vi "Tip Strip.vi"(7 "Calling VI's reference":refnum<vi>, 11 "Ref Array":refnum<vi>[](array[refnum])) -> ()   [LabVIEW 2017]
doc: "Registers events for array of references passed in. When a control is moused over, the tip strip text is shown in a popup as long as the mouse os over the control. The tip strip disappears when the mouse leaves the control or the mouse is clicked on the control.\n\nNEEDS: resize the tip strip to size of text."
uses:
  <vilib>/Utility/miscctls.llb/LVRectTypeDef.ctl
  <vilib>/Utility/inputDevices.llb/mouseAcquire.vi
panel:
  in  "Fade-Out Time [150]":u32=150
  in  "Fade-In Time [250]":u32=250
  out "error out":errorcluster
  in  "stop notifier":refnum<notifier>
  out "Custom Tip Strip":string
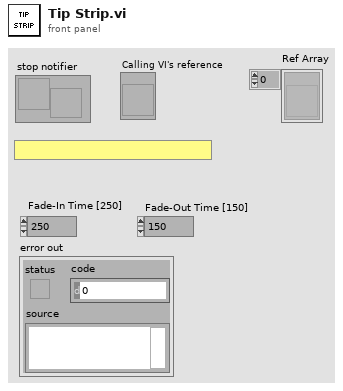
[diagram p1: front panel]
types:
  T1 = typedef "LVPositionTypeDef.ctl" = cluster{"Left":i32, "Top":i32}
  T2 = enum32{"Invalid", "Standard", "Closed", "Hidden", "Minimized", "Maximized"}
  T3 = cluster{"Font Name:":string, "Size":i16, "Strikeout?":bool, "Italic?":bool, "Underline?":bool, "Outline?":bool, "Shadow?":bool, "Bold?":bool}
  T4 = typedef "LVRectTypeDef.ctl" = cluster{"Left":i16, "Top":i16, "Right":i16, "Bottom":i16}
  T5 = cluster{"left":i16, "top":i16, "right":i16, "bottom":i16}
  T6 = cluster{"Horizontal":i32, "Vertical":i32, "Scrolling":i32}
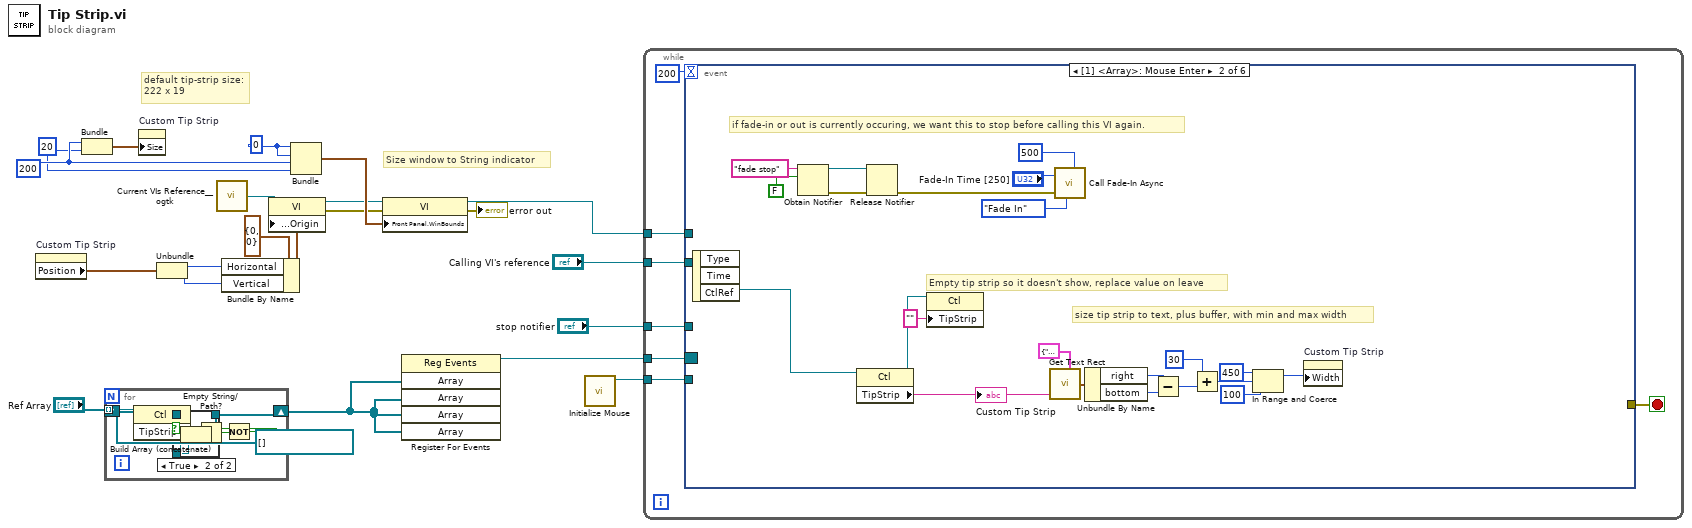
[diagram p0: block diagram]
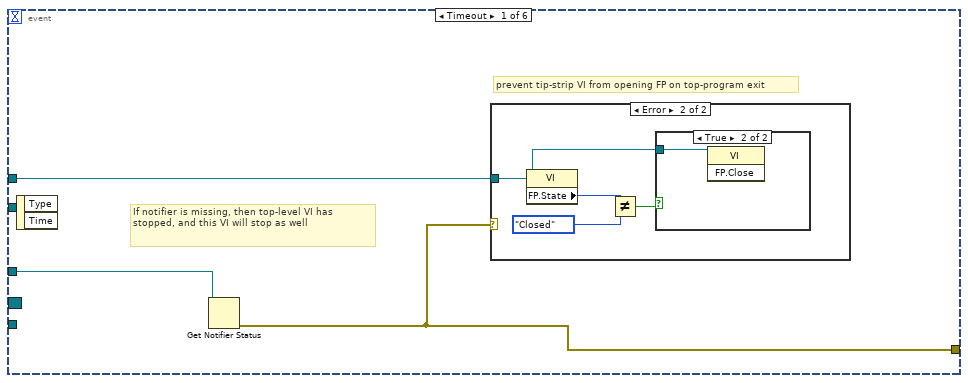
[diagram p3: hidden frame]
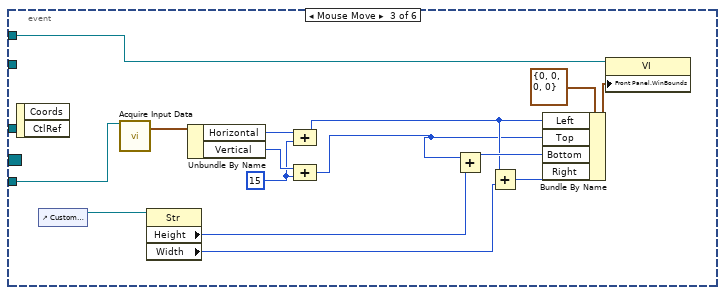
[diagram p6: hidden frame]
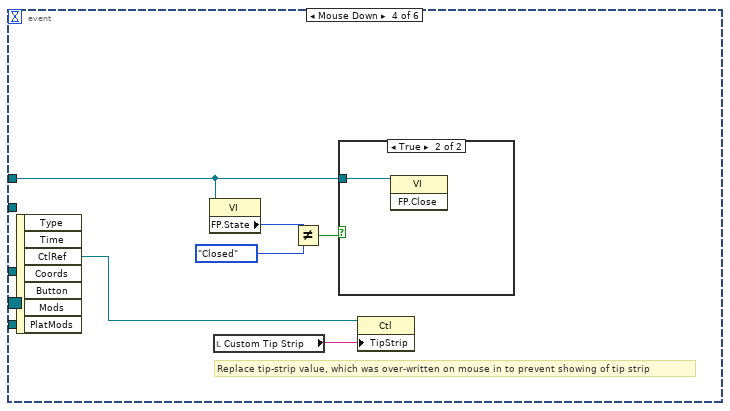
[diagram p7: hidden frame]
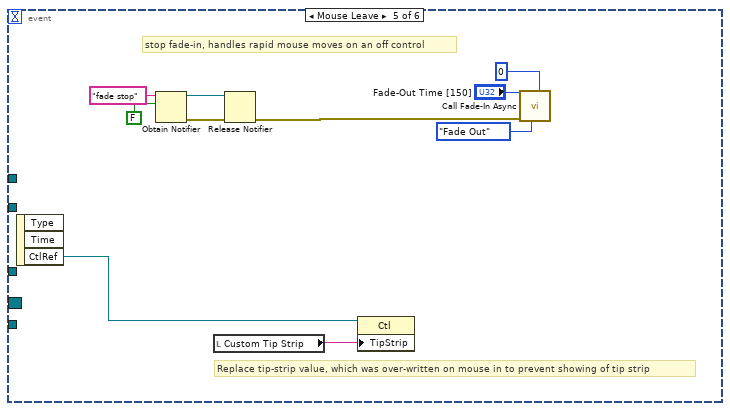
[diagram p9: hidden frame]
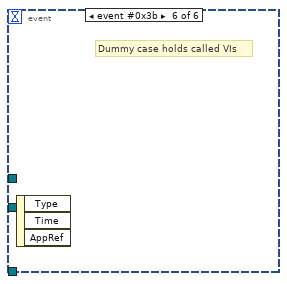
[diagram p10: hidden frame]
diagram:
  w2 = 20
  w3 = 200
  w8 = 0
  # "default tip-strip size:\n222 x 19"
  # "Size window to String indicator"
  n1 = property on="Custom Tip Strip" class="Str"() -> ("Position"=w19:T1)  [unwired: 2 in, 2 out]
  n2 = Bundle(w3, w2) -> (w4:cluster{i32, i32})  [unwired: 1 in]
  n3 = for {
    tunnel: "Ref Array" -> [w29] mode=indexing
    shift-right: [w23] -> w5
    shift-left: refnum<vi>[] [] ("Array") -> [w24]
    n4 = property class="Ctl"(reference=w29) -> (reference out=w28:refnum<vi>, "TipStrip"=w27:string)  [unwired: 1 in, 1 out]
    n5 = Empty String/Path?(string/path=w27) -> (empty?=w26:bool)
    n6 = Not(x=w26) -> (.not. x?=w25:bool)
    n7 = case shown="True" w25 {
      tunnel: w24 -> [w30 w32]
      tunnel: w28 -> [_ w31]
      tunnel: [w30 w33] -> w23
      frame False {
      }
      frame True {
        n8 = Build Array (concatenate)(w32, w31) -> (w33:refnum<vi>[])
      }
    }
  }
  n9 = property on="Custom Tip Strip" class="Str"("Size"=w4) -> ()  [unwired: 2 in, 2 out]
  n10 = Unbundle(w19) -> ("Left"=w11:i32, "Top"=w10:i32)
  n11 = call "Current VIs Reference__ogtk.vi"() -> ("Current VI's reference"=w12:refnum<vi>)  [unwired: 5 in]
  n12 = Bundle By Name(cluster=cluster{"Horizontal":i16, "Vertical":i16} {"Horizontal"=0, "Vertical"=0} ("Front Panel Window:Origin"), "Horizontal"=w11, "Vertical"=w10) -> (w14:cluster{"Horizontal":i16, "Vertical":i16})
  n13 = property on="Property Node" class="VI"(reference=w12, "Front Panel Window:Origin"=w14) -> (reference out=w13:refnum<vi>, error out=w9:errorcluster)  [unwired: 1 in]
  n14 = Bundle(w8, w8, w3, w2) -> (w18:cluster{i32, i32, i32, i32})  [unwired: 1 in]
  n15 = property class="VI"(reference=w13, error in=w9, "Front Panel.WinBounds"=w18) -> (reference out=w17:refnum<vi>, error out=→"error out":errorcluster)
  n16 = register-events(w5, w5, w5, w5) -> (reference out=w22:refnum<event-registration>)  [unwired: 2 in, 1 out]
  n17 = call <vilib>:"Initialize Mouse.vi"() -> ("device ID"=w7:refnum<k1>)  [unwired: 10 in, 1 out]
  n18 = while {
    tunnel: w22 -> [w40]
    tunnel: w17 -> [w38]
    tunnel: "stop notifier" -> [w37]
    tunnel: "Calling VI's reference" -> [w35]
    tunnel: w7 -> [w34]
    stop <- w39 stop-if-true
    n19 = event shown="[1] <Array>: Mouse Enter" {
      selector: w40 -> [_ _ _ _ _ _]
      dyn-events: _ -> [_ _ _ _ _ _]
      timeout: 200 -> [_ _ _ _ _ _]
      tunnel: [w42 _ _ _ _ _] -> w39
      tunnel: w38 -> [w41 _ w76 w91 _ _]
      tunnel: w37 -> [w43 _ _ _ _ _]
      tunnel: w35 -> [_ _ _ _ _ _]
      tunnel: w34 -> [_ _ w83 _ _ _]
      event Timeout {
        # "prevent tip-strip VI from opening FP on top-program exit"
        # "If notifier is missing, then top-level VI has stopped, and this VI will stop as well"
        n20 = event-data() -> ()  [unwired: 1 in, 2 out]
        n21 = Get Notifier Status(notifier=w43) -> (error out=w42:errorcluster)  [unwired: 1 in, 4 out]
        n22 = case shown="Error" w42 {
          tunnel: w41 -> [_ w44]
          frame No Error {
          }
          frame Error {
            n23 = property class="VI"(reference=w44) -> ("FP.State"=w47:T2)  [unwired: 1 in, 2 out]
            n24 = Not Equal?(x=w47, y=T2."Closed" ("Front Panel Window:State")) -> (x != y?=w45:bool)
            n25 = case shown="True" w45 {
              tunnel: w44 -> [_ w48]
              frame False {
              }
              frame True {
                n26 = invoke class="VI" method="FP.Close"(reference=w48) -> ()  [unwired: 2 in, 3 out]
              }
            }
          }
        }
      }
      event Mouse Enter {
        # "if fade-in or out is currently occuring, we want this to stop before calling this VI again."
        # "size tip strip to text, plus buffer, with min and max width"
        # "Empty tip strip so it doesn't show, replace value on leave"
        n27 = event-data() -> ("CtlRef"=w70:refnum<vi>)  [unwired: 1 in, 2 out]
        n28 = Obtain Notifier(name (unnamed)="fade stop", notification data type=FALSE) -> (notifier out=w50:refnum<notifier>, error out=w51:errorcluster)  [unwired: 2 in, 1 out]
        n29 = property class="Ctl"(reference=w70) -> (reference out=w58:refnum<vi>, "TipStrip"=w57:string)  [unwired: 1 in, 1 out]
        "Custom Tip Strip" <- w57
        n30 = Release Notifier(notifier=w50, error in (no error)=w51) -> (error out=w49:errorcluster)  [unwired: 1 in, 2 out]
        n31 = property class="Ctl"(reference=w58, "TipStrip"="" ("Tip Strip")) -> ()  [unwired: 1 in, 2 out]
        n32 = call <vilib>:"Get Text Rect.vi"("text"=w57, "[user-specified font]"=T3 {"Font Name:"="", "Size"=15, "Strikeout?"=FALSE, "Italic?"=FALSE, "Underline?"=FALSE, "Outline?"=FALSE, "Shadow?"=FALSE, "Bold?"=FALSE}) -> ("rect"=w69:T5)  [unwired: 7 in]
        n33 = call "Call Fade-In Async.vi"("Delay (ms) [0]"=500, "Fade Direction [Fade In]"=enum16{"Fade In", "Fade Out"}."Fade In", "Fade-In Time (ms)"="Fade-In Time [250]", "error in (no error)"=w49) -> ()  [unwired: 7 in, 1 out]
        n34 = Unbundle By Name(w69) -> ("right"=w68:i16, "bottom"=w67:i16)
        n35 = Subtract(x=w68, y=w67) -> (x-y=w65:i16)
        n36 = Add(x=30, y=w65) -> (x+y=w63:i32)
        n37 = In Range and Coerce(upper limit=450, x=w63, lower limit=100) -> (coerced(x)=w60:i32)  [unwired: 1 out]
        n38 = property on="Custom Tip Strip" class="Str"("Width"=w60) -> ()  [unwired: 2 in, 2 out]
      }
      event Mouse Move {
        w79 = 15
        n39 = event-data() -> ()  [unwired: 1 in, 2 out]
        n40 = control-ref of="Custom Tip Strip"() -> (w75:refnum<vi>)
        n41 = call-poly <vilib>:"Acquire Input Data.vi"("device ID"=w83) -> ("axis info"=w82:T6)  [unwired: 15 in, 3 out]
        n42 = property class="Str"(reference=w75) -> ("Height"=w74:u32, "Width"=w73:u32)  [unwired: 1 in, 2 out]
        n43 = Unbundle By Name(w82) -> ("Horizontal"=w81:i32, "Vertical"=w80:i32)
        n44 = Compound Arithmetic op=ADD(w81, w79) -> (w78:i32)
        n45 = Compound Arithmetic op=ADD(w80, w79) -> (w77:i32)
        n46 = Add(x=w77, y=w74) -> (x+y=w85:u32)
        n47 = Add(x=w78, y=w73) -> (x+y=w84:u32)
        n48 = Bundle By Name(cluster=T4 {"Left"=0, "Top"=0, "Right"=0, "Bottom"=0} ("Front Panel Window:Window Bounds"), "Left"=w78, "Top"=w77, "Bottom"=w85, "Right"=w84) -> (w72:T4)
        n49 = property class="VI"(reference=w76, "Front Panel.WinBounds"=w72) -> ()  [unwired: 1 in, 2 out]
      }
      event Mouse Down {
        # "Replace tip-strip value, which was over-written on mouse in to prevent showing of tip strip"
        n50 = event-data() -> ("CtlRef"=w90:refnum<vi>)  [unwired: 1 in, 6 out]
        n51 = property class="VI"(reference=w91) -> ("FP.State"=w88:T2)  [unwired: 1 in, 2 out]
        n52 = local read "Custom Tip Strip"() -> (w89:string)
        n53 = Not Equal?(x=w88, y=T2."Closed" ("Front Panel Window:State")) -> (x != y?=w86:bool)
        n54 = case shown="True" w86 {
          tunnel: w91 -> [_ w92]
          frame False {
          }
          frame True {
            n55 = invoke class="VI" method="FP.Close"(reference=w92) -> ()  [unwired: 2 in, 3 out]
          }
        }
        n56 = property class="Ctl"(reference=w90, "TipStrip"=w89) -> ()  [unwired: 1 in, 2 out]
      }
      event Mouse Leave {
        # "stop fade-in, handles rapid mouse moves on an off control"
        # "Replace tip-strip value, which was over-written on mouse in to prevent showing of tip strip"
        n57 = event-data() -> ("CtlRef"=w102:refnum<vi>)  [unwired: 1 in, 2 out]
        n58 = Obtain Notifier(name (unnamed)="fade stop", notification data type=FALSE) -> (notifier out=w94:refnum<notifier>, error out=w95:errorcluster)  [unwired: 2 in, 1 out]
        n59 = local read "Custom Tip Strip"() -> (w101:string)
        n60 = Release Notifier(notifier=w94, error in (no error)=w95) -> (error out=w93:errorcluster)  [unwired: 1 in, 2 out]
        n61 = property class="Ctl"(reference=w102, "TipStrip"=w101) -> ()  [unwired: 1 in, 2 out]
        n62 = call "Call Fade-In Async.vi"("Delay (ms) [0]"=0, "Fade Direction [Fade In]"=enum16{"Fade In", "Fade Out"}."Fade Out", "Fade-In Time (ms)"="Fade-Out Time [150]", "error in (no error)"=w93) -> ()  [unwired: 7 in, 1 out]
      }
      event event #0x3b {
        # "Dummy case holds called VIs"
        n63 = event-data() -> ()  [unwired: 1 in, 3 out]
      }
    }
  }
